vi "Get Angstrom Exponent.vi"(8 "error in (no error)":errorcluster, 10 "lambda":dbl[](array[numeric]), 11 "Extinction":dbl[](array[numeric])) -> (0 "error out":errorcluster, 2 "PlotData":T1(graph), 3 "AngstromExp":dbl)   [LabVIEW 2016, in "Atmospheric Library.lvlib"]
uses:
  Atmospheric Library.lvlib
  <vilib>/Analysis/NI_AALPro.lvlib
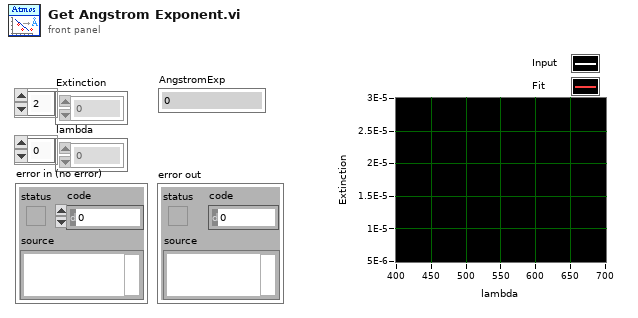
[diagram p1: front panel]
types:
  T1 = cluster{"lambda":dbl[], "Best Power Fit":dbl[]}[]
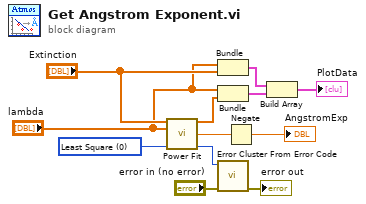
[diagram p0: block diagram]
diagram:
  w12 = u16 0 items=["Least Square", "Least Absolute Residual", "Bisquare"] ("method")
  n1 = call <vilib>:"Power Fit.vi"("Y"="Extinction", "X"="lambda", "method"=w12) -> ("Best Power Fit"=w8:dbl[], "power"=w2:dbl, "error"=w11:i32)  [unwired: 3 in, 7 out]
  n2 = Bundle("lambda"="lambda", "Extinction"="Extinction") -> (w7:cluster{"lambda":dbl[], "Extinction":dbl[]})  [unwired: 1 in]
  n3 = Bundle("lambda"="lambda", "Best Power Fit"=w8) -> (w6:cluster{"lambda":dbl[], "Best Power Fit":dbl[]})  [unwired: 1 in]
  n4 = call <vilib>:"Error Cluster From Error Code.vi"("error in (no error)"="error in (no error)", "error code (0)"=w11) -> ("error out"=→"error out":errorcluster)  [unwired: 7 in]
  n5 = Negate(x=w2) -> (-x=→"AngstromExp":dbl)
  n6 = Build Array(w7, w6) -> (→"PlotData":T1)
